vi "on-off controller setpoint 1.vi"(4 "State":i16, 5 "Time":dbl format="%.2f", 6 "Sensor Values":dbl[](array[numeric]), 7 "Set Points":dbl[](array[numeric])) -> (0 "required data":T1={"Set Point names"=["off value", "on value", "minimum target", "maximum target", "sensor"], "required number of setpoints"=5, "required number of sensors"=0, "Sensor names"=[]}, 3 "output value":dbl)   [LabVIEW 2019]
panel:
  # "Enter the correct information for this control code in the required data structure below. Then make the current value default by right clicking on the border of the data structure. Select \"data operations\" and then select \"make current value default\". These values will be displayed by process controller."
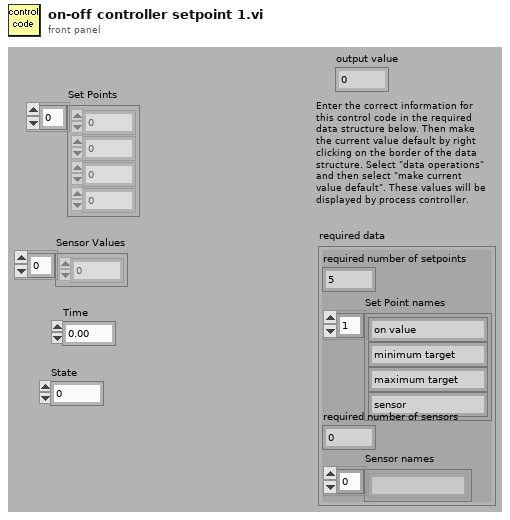
[diagram p1: front panel]
types:
  T1 = cluster{"Set Point names":string[], "required number of setpoints":u8, "required number of sensors":u8, "Sensor names":string[]}
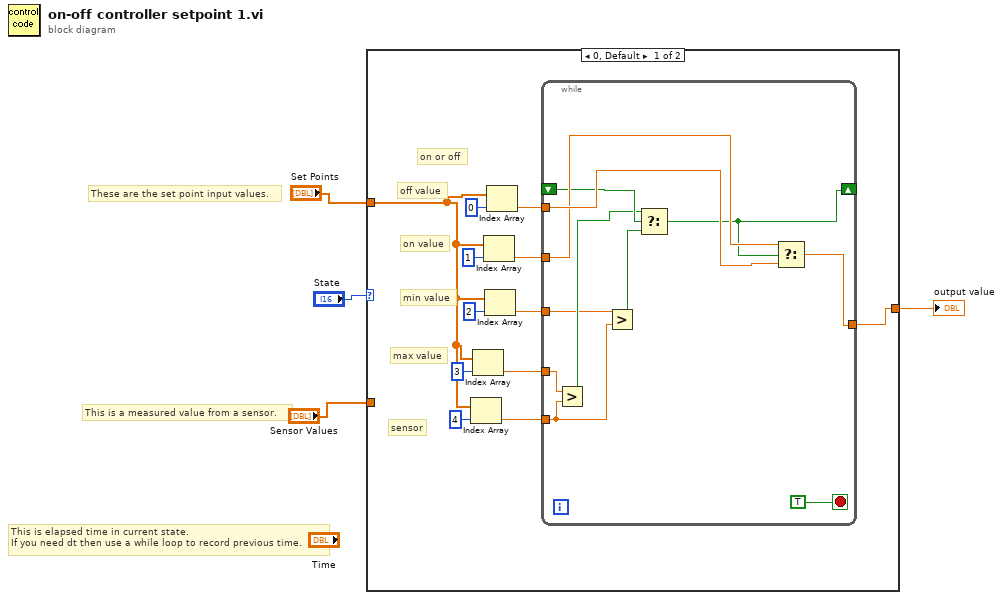
[diagram p0: block diagram]
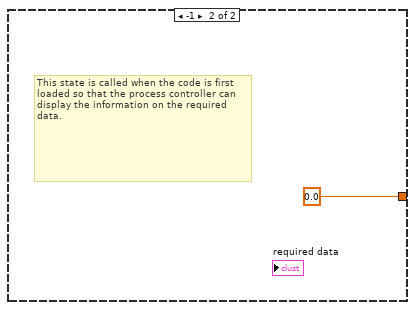
[diagram p2: hidden frame]
diagram:
  # "These are the set point input values."
  # "This is a measured value from a sensor."
  # "This is elapsed time in current state.\nIf you need dt then use a while loop to record previous time."
  n1 = case shown="0, Default" "State" {
    tunnel: [w10 0.0 ("fraction on")] -> w3
    tunnel: "Set Points" -> [w5 _]
    tunnel: "Sensor Values" -> [_ _]
    frame 0, Default {
      # "on value"
      # "on or off"
      # "sensor"
      # "min value"
      # "max value"
      # "off value"
      n2 = Index Array(array=w5, index=4) -> (element=w8:dbl)
      n3 = Index Array(array=w5, index=3) -> (element=w13:dbl)
      n4 = Index Array(array=w5, index=1) -> (element=w11:dbl)
      n5 = Index Array(array=w5, index=2) -> (element=w15:dbl)
      n6 = Index Array(array=w5, index=0) -> (element=w6:dbl)
      n7 = while {
        tunnel: w15 -> [w19]
        tunnel: w13 -> [w26]
        tunnel: w11 -> [w24]
        tunnel: [w23] -> w10
        tunnel: w8 -> [w18]
        tunnel: w6 -> [w25]
        shift-right: [w20] -> _
        shift-left: _ -> [w22]
        stop <- TRUE stop-if-true
        n8 = Greater?(x=w26, y=w18) -> (0:w21:bool)
        n9 = Greater?(x=w19, y=w18) -> (0:w17:bool)
        n10 = Select(t=w21, s=w22, f=w17) -> (s? t:f=w20:bool)
        n11 = Select(t=w24, s=w20, f=w25) -> (s? t:f=w23:dbl)
      }
    }
    frame -1 {
      # "This state is called when the code is first loaded so that the process controller can display the information on the required data."
    }
  }
  "output value" <- w3
